vi "Periodic Tasks.vi"(8 "error in":errorcluster) -> ()   [LabVIEW 2015]
doc: "This VI runs in parallel to other tasks. It can contain as many user-defined periodic loops as you need. These can carry out PID or other sorts of timed response."
uses:
  <vilib>/Rock Robotics/WPI/Utilities/WPI_GetSetVariantRefNum.vi
  Robot Global Data.vi
  <vilib>/Rock Robotics/Network Tables/NT Write Numeric Array.vi
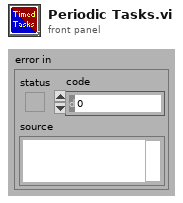
[diagram p1: front panel]
types:
  T1 = typedef "WPI_RobotDriveDevRef.ctl" = cluster{"DevStatus":errorcluster, "Motors[]":T2[], "Square Inputs":bool, "Max Output":dbl}
  T2 = typedef "WPI_MotorControlDeviceRef.ctl" = cluster{"DeviceStatus":errorcluster, "Type":T3, "PWM":cluster{"PWM Channel":T4, "DeadBand":T5}, "CAN":cluster{"Device Number":u8, "Control Mode":T6, "Semaphore":T7, "Max Vout":dbl, "TalonSRX Control Mode":T8}, "Invert":bool}
  T3 = typedef "WPI_MotorControlType.ctl" = enum16{"PWM", "CAN", "CANTalonSRX"}
  T4 = typedef "FPGA_DIOPWMChannel.ctl" = enum8{"PWM 0", "PWM 1", "PWM 2", "PWM 3", "PWM 4", "PWM 5", "PWM 6", "PWM 7", "PWM 8", "PWM 9", "PWM MXP 0", "PWM MXP 1", "PWM MXP 2", "PWM MXP 3", "PWM MXP 4", "PWM MXP 5", "PWM MXP 6", "PWM MXP 7", "PWM MXP 8", "PWM MXP 9", "Invalid"}
  T5 = typedef "WPI_PWMDeadband.ctl" = cluster{"Name":string, "maxPositivePwm":i32, "minPositivePwm":i32, "centerPwm":i32, "maxNegativePwm":i32, "minNegativePwm":i32, "angularRange":u16}
  T6 = typedef "WPI_CANJaguar_ControlMode.ctl" = enum8{"Percent VBus", "Current", "Speed", "Position", "Voltage"}
  T7 = typedef "Semaphore RefNum" = refnum<k1>
  T8 = typedef "WPI_CANTalonSRX_APIControlMode.ctl" = enum8{"Percent VBus", "Speed", "Position", "Slave", "Unchanged / Invalid", "Voltage Compensation", "Current", "Motion Profile"}
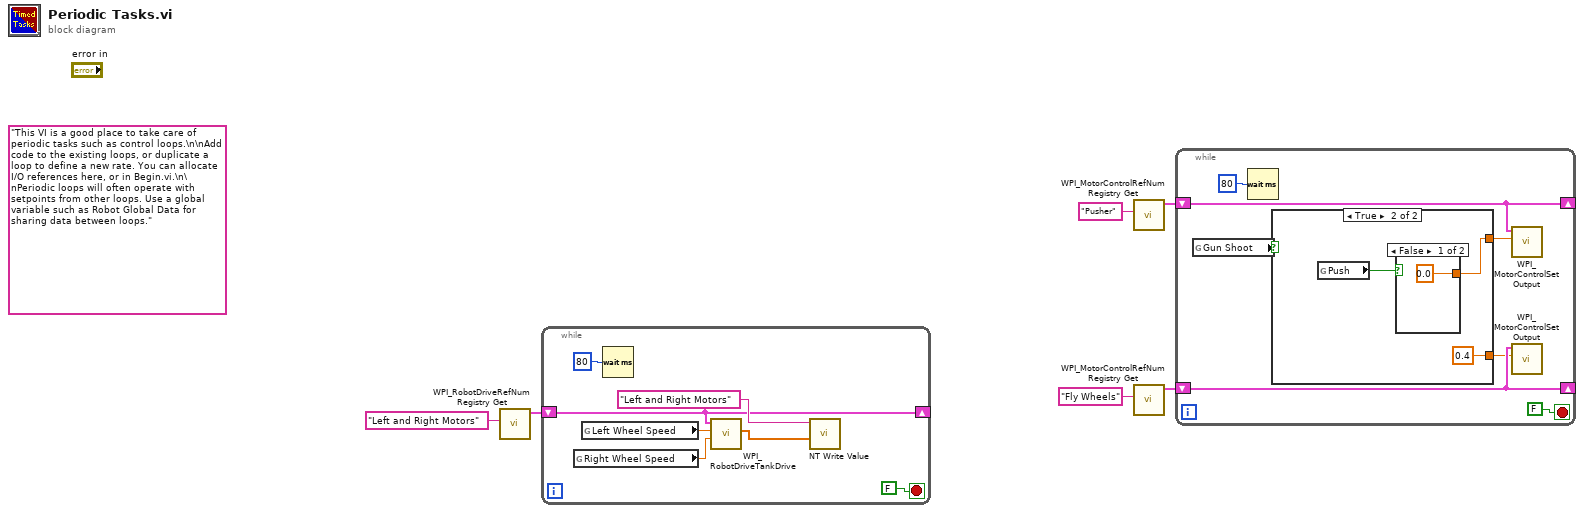
[diagram p0: block diagram]
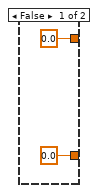
[diagram p2: hidden frame]
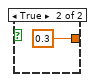
[diagram p3: hidden frame]
diagram:
  (unwired) "This VI is a good place to take care of periodic tasks such as control loops.\n\nAdd code to the existing loops, or duplicate a loop to define a new rate. You can allocate I/O references here, or in Begin.vi.\n\nPeriodic loops will often operate with setpoints from other loops. Use a global variable such as Robot Global Data for sharing data between loops."
  n1 = call <vilib>:"WPI_RobotDriveRefNum Registry Get.vi"("refnum name"="Left and Right Motors") -> ("RobotDriveDevRef"=w5:T1)  [unwired: 1 in, 9 out]
  n2 = while {
    shift-right: [w11] -> _
    shift-left: w5 -> [w11]
    stop <- FALSE stop-if-true
    n3 = global read "Robot Global Data.vi" "Right Wheel Speed"() -> (w9:dbl)
    n4 = global read "Robot Global Data.vi" "Left Wheel Speed"() -> (w10:dbl)
    n5 = Wait (ms)(milliseconds to wait=u32 80) -> ()  [unwired: 1 out]
    n6 = call <vilib>:"WPI_RobotDriveTankDrive.vi"("Right axis value"=w9, "Left axis value"=w10, "RobotDriveDevRef"=w11) -> ("Motor Values"=w13:dbl[])  [unwired: 6 in, 2 out]
    n7 = call-poly <vilib>:"NT Write Value.vi"("Numeric Array"=w13, "Name"="Left and Right Motors") -> ()  [unwired: 9 in, 1 out]
  }
  n8 = call <vilib>:"WPI_MotorControlRefNum Registry Get.vi"("refnum name"="Pusher") -> ("MotorControlDevRef"=w1:T2)  [unwired: 9 in, 1 out]
  n9 = call <vilib>:"WPI_MotorControlRefNum Registry Get.vi"("refnum name"="Fly Wheels") -> ("MotorControlDevRef"=w3:T2)  [unwired: 9 in, 1 out]
  n10 = while {
    shift-right: [w20] -> _
    shift-left: w3 -> [w20]
    shift-right: [w15] -> _
    shift-left: w1 -> [w15]
    stop <- FALSE stop-if-true
    n11 = global read "Robot Global Data.vi" "Gun Shoot"() -> (w19:bool)
    n12 = Wait (ms)(milliseconds to wait=u32 80) -> ()  [unwired: 1 out]
    n13 = case shown="True" w19 {
      tunnel: [0.0 ("Output") 0.4 ("Output")] -> w18
      tunnel: [0.0 ("Output") w23] -> w14
      frame False {
      }
      frame True {
        n14 = global read "Robot Global Data.vi" "Push"() -> (w24:bool)
        n15 = case shown="False" w24 {
          tunnel: [0.0 ("Output") 0.3 ("Output")] -> w23
          frame False {
          }
          frame True {
          }
        }
      }
    }
    n16 = call <vilib>:"WPI_MotorControlSetOutput.vi"("Output"=w14, "MotorControlDevRef"=w15) -> ()  [unwired: 7 in, 3 out]
    n17 = call <vilib>:"WPI_MotorControlSetOutput.vi"("Output"=w18, "MotorControlDevRef"=w20) -> ()  [unwired: 7 in, 3 out]
  }
